vi "DAQ - Reserve Device.vi"(11 "device in":tag) -> (0 "error out":errorcluster, 3 "device out":tag)   [LabVIEW 2021]
doc: "Reserves a device with DAQmx and provides a screen alerting user to wait."
panel:
  # "Attempting to reserve cDAQ, please wait."
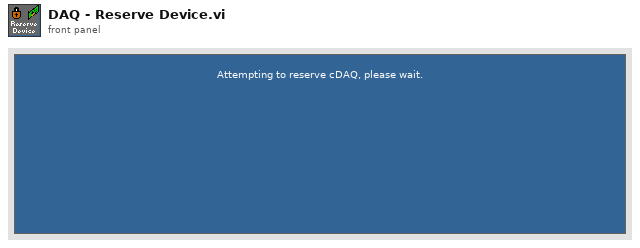
[diagram p1: front panel]
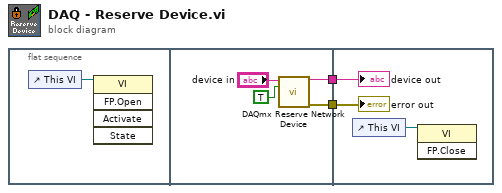
[diagram p0: block diagram]
diagram:
  n1 = flat-sequence {
    tunnel: [w5] -> w2
    tunnel: [w4] -> w1
    tunnel: w2 -> [w10]
    tunnel: w1 -> [w9]
    frame #0 {
      n2 = control-ref of="This VI"() -> (w3:refnum<vi>)
      n3 = invoke class="VI" method="FP.Open"(reference=w3) -> ()  [unwired: 4 in, 5 out]
    }
    frame #1 {
      n4 = call <vilib>:"DAQmx Reserve Network Device.vi"("device in"="device in", "override reservation?"=TRUE) -> ("device out"=w4:tag, "error out"=w5:errorcluster)  [unwired: 12 in]
    }
    frame #2 {
      n5 = control-ref of="This VI"() -> (w8:refnum<vi>)
      n6 = invoke class="VI" method="FP.Close"(reference=w8) -> ()  [unwired: 2 in, 3 out]
      "error out" <- w10
      "device out" <- w9
    }
  }
